vi "Emailer Handler Open Config.vi"(10 "Config Path":path, 11 "Emails IN":T1[](array[typedef])) -> (3 "Emails OUT":T1[](array[typedef]))   [LabVIEW 2019]
uses:
  Type Defs/Email Cluster v2.ctl
  Type Defs/Email Cluster v1.ctl
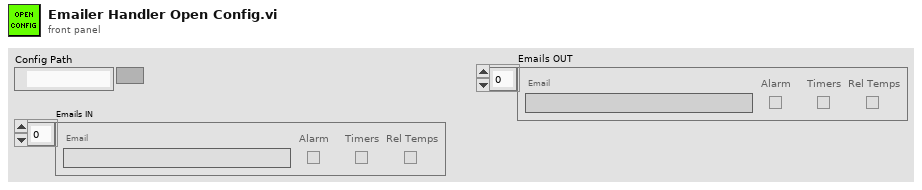
[diagram p1: front panel]
types:
  T1 = typedef "Email Cluster v2.ctl" = cluster{"Email":string, "Alarm":bool, "Timers":bool, "Rel Temps":bool}
  T2 = typedef "Email Cluster v1.ctl" = cluster{"Email":string, "Alarm":bool, "Timers":bool}
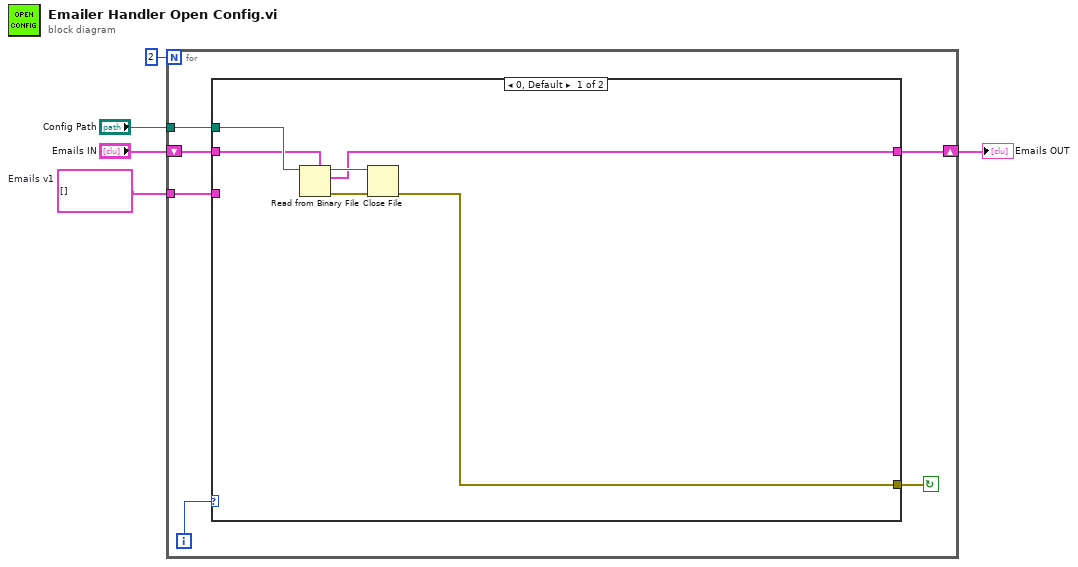
[diagram p0: block diagram]
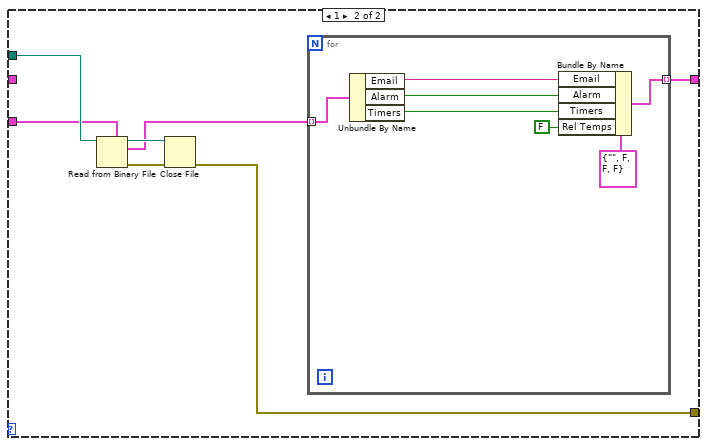
[diagram p2: hidden frame]
diagram:
  w1 = T2[] []  # Emails v1
  n1 = for {
    N: 2 -> [_]
    tunnel: w1 -> [w9]
    tunnel: "Config Path" -> [w8]
    shift-right: [w6] -> w2
    shift-left: "Emails IN" -> [w10]
    i -> [w11]
    stop <- w7 continue-if-true
    n2 = case shown="0, Default" w11 {
      tunnel: w10 -> [w16 _]
      tunnel: w9 -> [_ w20]
      tunnel: w8 -> [w17 w24]
      tunnel: [w13 w21] -> w7
      tunnel: [w12 w19] -> w6
      frame 0, Default {
        n3 = Read from Binary File(5:w16, 11:w17) -> (0:w14:errorcluster, 2:w12:T1[], 3:w15:refnum<file>)  [unwired: 4 in, 1 out]
        n4 = Close File(refnum=w15, error in=w14) -> (error out=w13:errorcluster)  [unwired: 1 out]
      }
      frame 1 {
        n5 = Read from Binary File(5:w20, 11:w24) -> (0:w22:errorcluster, 2:w18:T2[], 3:w23:refnum<file>)  [unwired: 4 in, 1 out]
        n6 = Close File(refnum=w23, error in=w22) -> (error out=w21:errorcluster)  [unwired: 1 out]
        n7 = for {
          tunnel: w18 -> [w30] mode=indexing
          tunnel: [w25] -> w19 mode=indexing
          n8 = Unbundle By Name(w30) -> ("Email"=w29:string, "Alarm"=w28:bool, "Timers"=w27:bool)
          n9 = Bundle By Name(cluster=T1 {"Email"="", "Alarm"=FALSE, "Timers"=FALSE, "Rel Temps"=FALSE} ("Email Cluster"), "Email"=w29, "Alarm"=w28, "Timers"=w27, "Rel Temps"=FALSE) -> (w25:T1)
        }
      }
    }
  }
  "Emails OUT" <- w2
